vi "output.vi"() -> ()   [LabVIEW 2019]
uses:
  <vilib>/Rock Robotics/WPI/ThirdParty/Phoenix-LabVIEW/Motor Controller/Controls/CTRE_Phoenix_MotorControl_ControlMode.ctl
  <vilib>/Rock Robotics/WPI/Utilities/WPI_GetSetVariantRefNum.vi
  <vilib>/Rock Robotics/Network Tables/NT Write Boolean Array.vi
  <vilib>/Rock Robotics/Network Tables/NT Write Numeric Array.vi
panel:
  in  "Output 5":T1 items=["PercentOutput"=0, "Position"=1, "Velocity"=2, "Current"=3, "Follower"=5, "MotionProfile"=6, "MotionMagic"=7, "MotionProfileArc"=10, "Disabled"=15]
  in  "Intake 4":T1 items=["PercentOutput"=0, "Position"=1, "Velocity"=2, "Current"=3, "Follower"=5, "MotionProfile"=6, "MotionMagic"=7, "MotionProfileArc"=10, "Disabled"=15]
  in  "Intake 3":T1 items=["PercentOutput"=0, "Position"=1, "Velocity"=2, "Current"=3, "Follower"=5, "MotionProfile"=6, "MotionMagic"=7, "MotionProfileArc"=10, "Disabled"=15]
  in  "Output 4":T1 items=["PercentOutput"=0, "Position"=1, "Velocity"=2, "Current"=3, "Follower"=5, "MotionProfile"=6, "MotionMagic"=7, "MotionProfileArc"=10, "Disabled"=15]
  in  "Output 3":T1 items=["PercentOutput"=0, "Position"=1, "Velocity"=2, "Current"=3, "Follower"=5, "MotionProfile"=6, "MotionMagic"=7, "MotionProfileArc"=10, "Disabled"=15]
  in  "Intake 2":T1 items=["PercentOutput"=0, "Position"=1, "Velocity"=2, "Current"=3, "Follower"=5, "MotionProfile"=6, "MotionMagic"=7, "MotionProfileArc"=10, "Disabled"=15]
  in  "Intake":T1 items=["PercentOutput"=0, "Position"=1, "Velocity"=2, "Current"=3, "Follower"=5, "MotionProfile"=6, "MotionMagic"=7, "MotionProfileArc"=10, "Disabled"=15]
  in  "Output":T1 items=["PercentOutput"=0, "Position"=1, "Velocity"=2, "Current"=3, "Follower"=5, "MotionProfile"=6, "MotionMagic"=7, "MotionProfileArc"=10, "Disabled"=15]
  in  "Intake":T1 items=["PercentOutput"=0, "Position"=1, "Velocity"=2, "Current"=3, "Follower"=5, "MotionProfile"=6, "MotionMagic"=7, "MotionProfileArc"=10, "Disabled"=15]
  in  "Output":T1 items=["PercentOutput"=0, "Position"=1, "Velocity"=2, "Current"=3, "Follower"=5, "MotionProfile"=6, "MotionMagic"=7, "MotionProfileArc"=10, "Disabled"=15]
  in  "Intake":T1 items=["PercentOutput"=0, "Position"=1, "Velocity"=2, "Current"=3, "Follower"=5, "MotionProfile"=6, "MotionMagic"=7, "MotionProfileArc"=10, "Disabled"=15]
  in  "Output 2":T1 items=["PercentOutput"=0, "Position"=1, "Velocity"=2, "Current"=3, "Follower"=5, "MotionProfile"=6, "MotionMagic"=7, "MotionProfileArc"=10, "Disabled"=15]
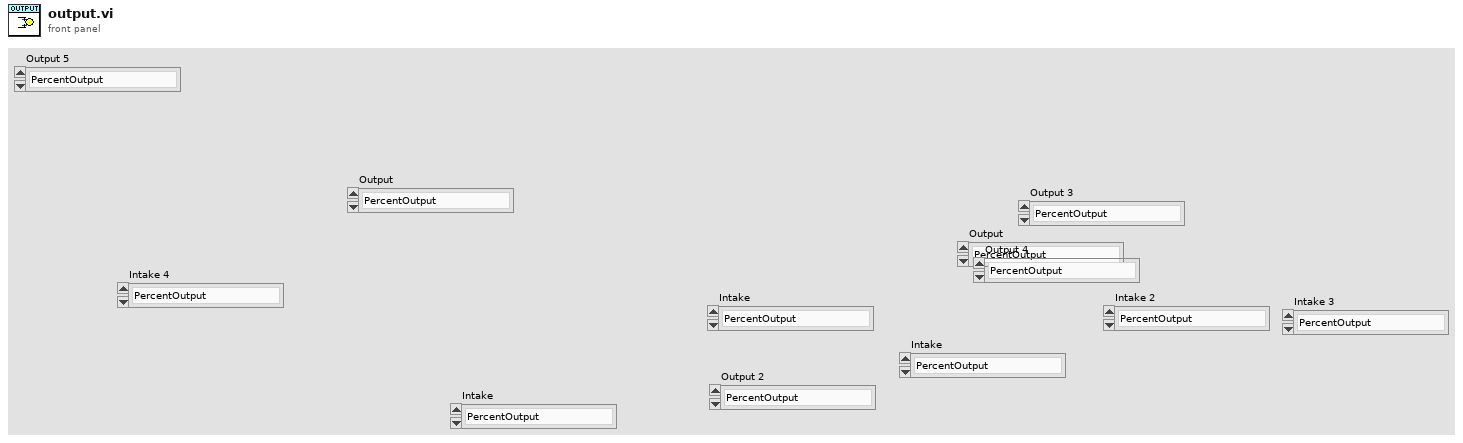
[diagram p1: front panel]
types:
  T1 = typedef "CTRE_Phoenix_MotorControl_ControlMode.ctl" = u16
  T2 = typedef "WPI_MotorControlDeviceRef.ctl" = cluster{"DeviceStatus":errorcluster, "Type":T3, "PWM":cluster{"PWM Channel":T4, "DeadBand":T5}, "CAN":cluster{"Device Number":u8, "SetOutput VI Ref":variant, "GetOutput VI Ref":variant, "Enable VI Ref":variant, "Disable VI Ref":variant, "Data":variant}, "Invert":bool, "DIO PWM":cluster{"PWM \"Enable\" Channel":T4, "DIOChannel":T6, "PWM Rate":dbl}}
  T3 = typedef "WPI_MotorControlType.ctl" = enum16{"PWM", "CAN", "DIO PWM"}
  T4 = typedef "FPGA_DIOPWMChannel.ctl" = enum8{"PWM 0", "PWM 1", "PWM 2", "PWM 3", "PWM 4", "PWM 5", "PWM 6", "PWM 7", "PWM 8", "PWM 9", "PWM MXP 0", "PWM MXP 1", "PWM MXP 2", "PWM MXP 3", "PWM MXP 4", "PWM MXP 5", "PWM MXP 6", "PWM MXP 7", "PWM MXP 8", "PWM MXP 9", "Invalid"}
  T5 = typedef "WPI_PWMDeadband.ctl" = cluster{"Name":string, "maxPositivePwm":i32, "minPositivePwm":i32, "centerPwm":i32, "maxNegativePwm":i32, "minNegativePwm":i32, "angularRange":u16}
  T6 = typedef "FPGA_DIOChannel.ctl" = enum8{"DIO 0", "DIO 1", "DIO 2", "DIO 3", "DIO 4", "DIO 5", "DIO 6", "DIO 7", "DIO 8", "DIO 9", "DIO MXP 0", "DIO MXP 1", "DIO MXP 2", "DIO MXP 3", "DIO MXP 4", "DIO MXP 5", "DIO MXP 6", "DIO MXP 7", "DIO MXP 8", "DIO MXP 9", "DIO MXP 10", "DIO MXP 11", "DIO MXP 12", "DIO MXP 13", "DIO MXP 14", "DIO MXP 15", "SPI Port CS1", "SPI Port CS2", "SPI Port CS3", "SPI Port MISO", "SPI Port MOSI", "Invalid"}
  T7 = typedef "WPI_JoystickDevRef.ctl" = cluster{"Device":T8}
  T8 = typedef "WPI_JoystickDeviceEnum.ctl" = enum16{"USB 0", "USB 1", "USB 2", "USB 3", "USB 4", "USB 5"}
  T9 = enum16{"Output Motor On", "Intake Motor On", "Complete"}
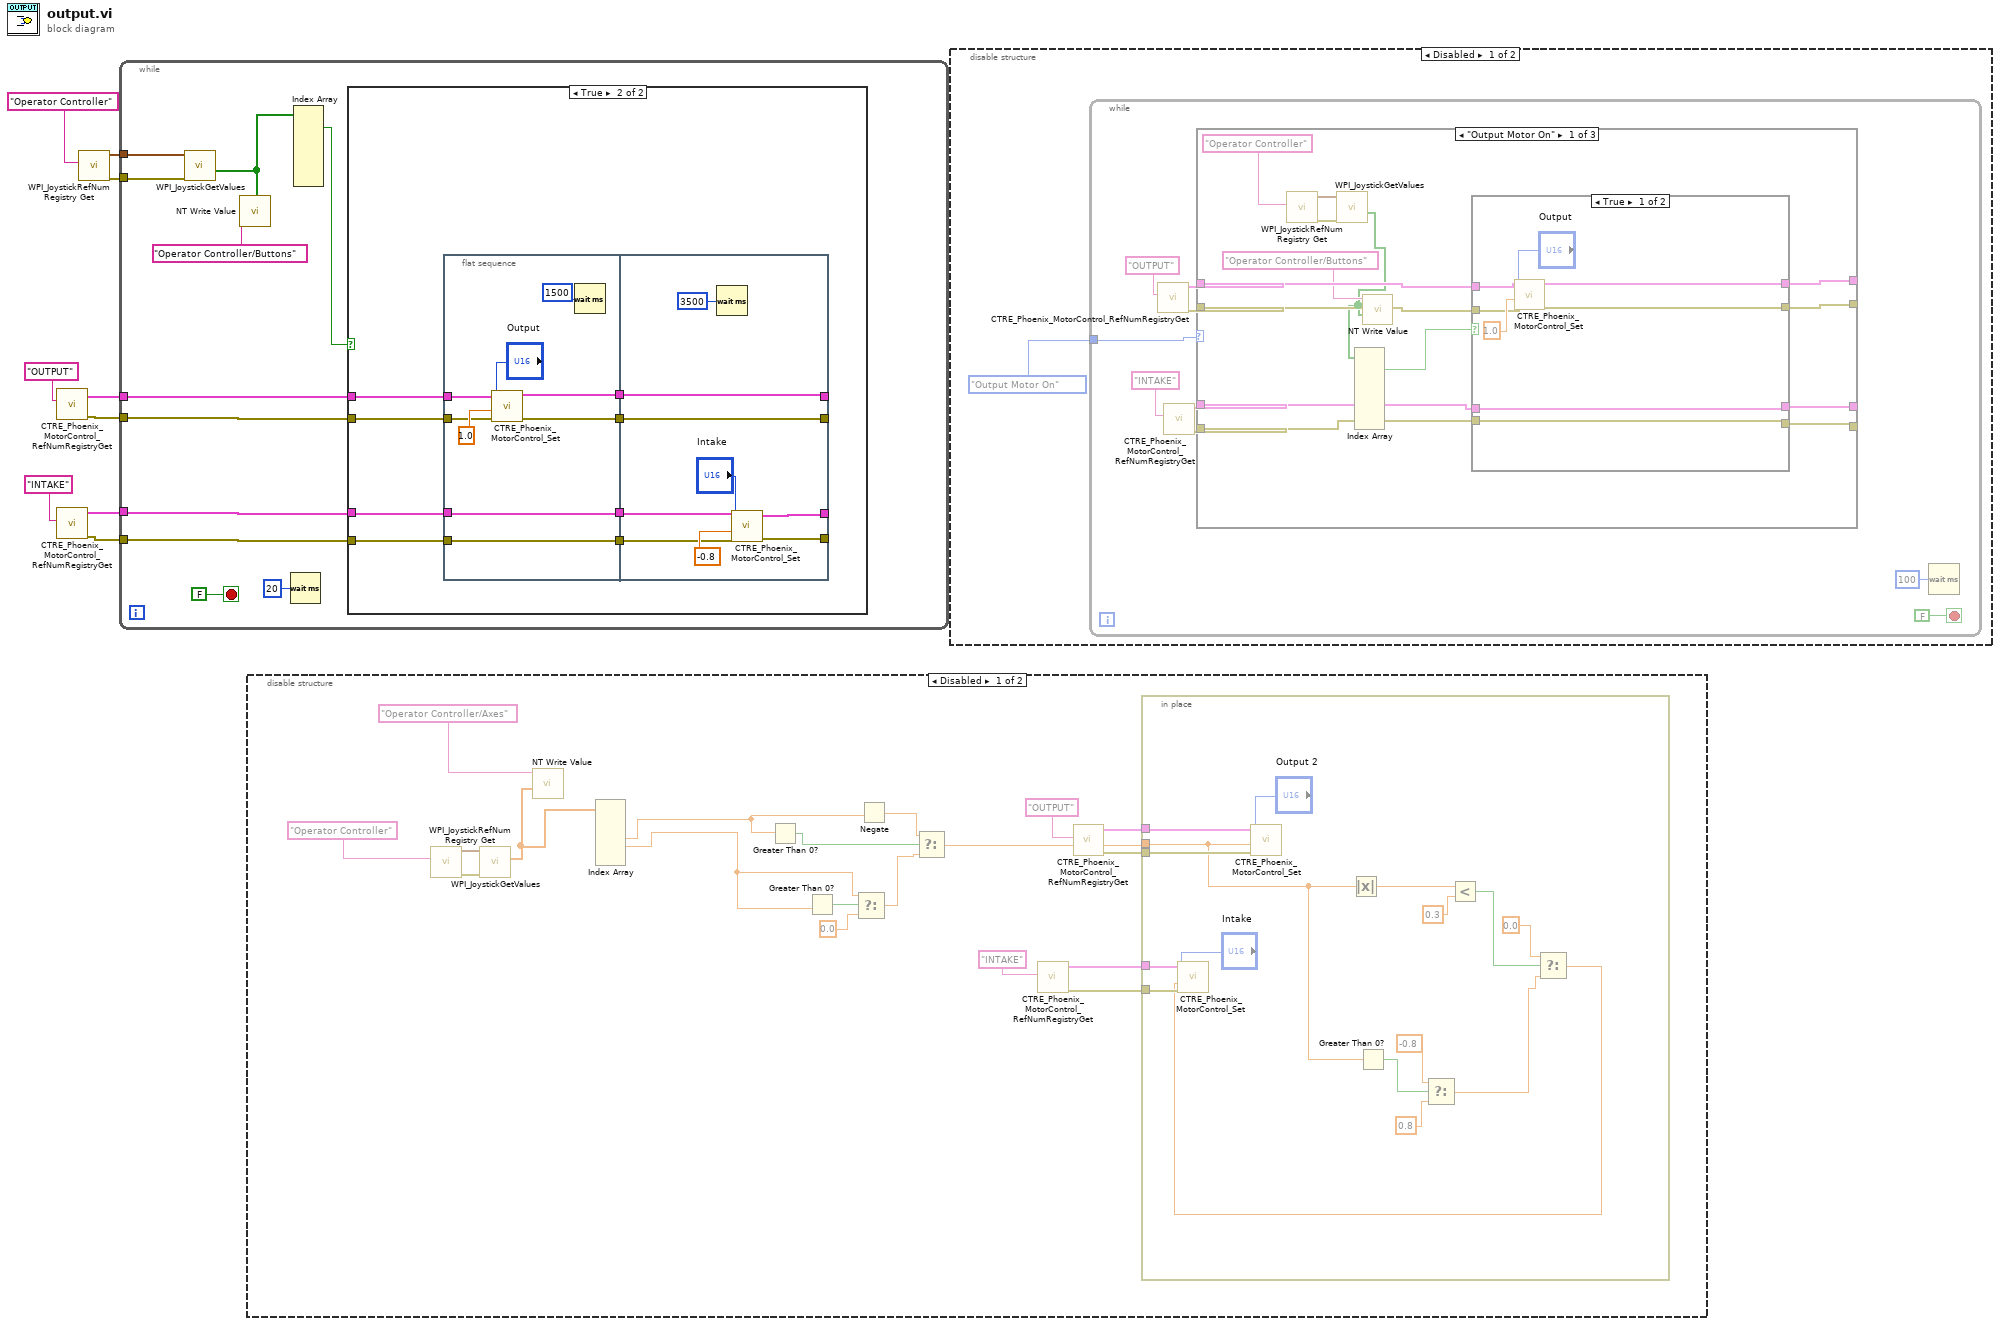
[diagram p0: block diagram]
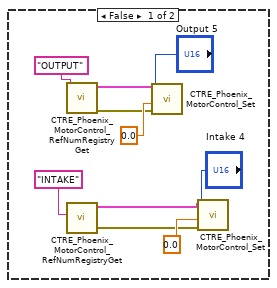
[diagram p2: hidden frame]
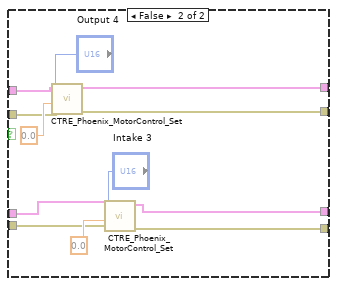
[diagram p3: hidden frame]
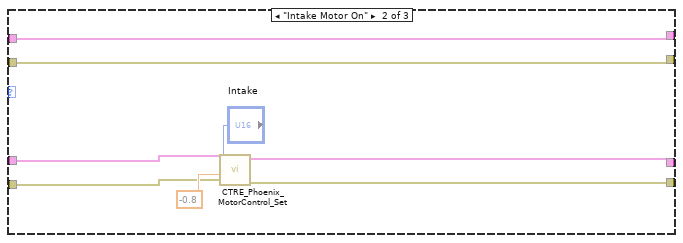
[diagram p4: hidden frame]
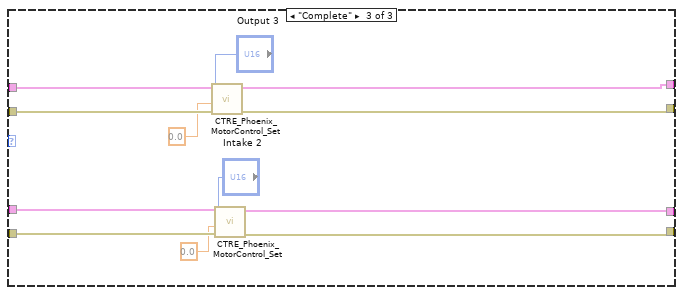
[diagram p5: hidden frame]
diagram:
  n1 = call <vilib>:"CTRE_Phoenix_MotorControl_RefNumRegistryGet.vi"("refnum name"="OUTPUT") -> ("error out"=w2:errorcluster, "PhoenixMotorControlDevRef"=w1:T2)  [unwired: 9 in]
  n2 = call <vilib>:"CTRE_Phoenix_MotorControl_RefNumRegistryGet.vi"("refnum name"="INTAKE") -> ("error out"=w4:errorcluster, "PhoenixMotorControlDevRef"=w3:T2)  [unwired: 9 in]
  n3 = call <vilib>:"WPI_JoystickRefNum Registry Get.vi"("refnum name"="Operator Controller") -> ("error out"=w7:errorcluster, "JoystickDevRef"=w8:T7)  [unwired: 1 in, 8 out]
  n4 = while {
    tunnel: w8 -> [w20]
    tunnel: w7 -> [w19]
    tunnel: w4 -> [w15]
    tunnel: w3 -> [w14]
    tunnel: w2 -> [w13]
    tunnel: w1 -> [w12]
    stop <- FALSE stop-if-true
    n5 = call <vilib>:"WPI_JoystickGetValues.vi"("error in (no error)"=w19, "JoystickDevRef"=w20) -> ("Buttons"=w17:bool[])  [unwired: 5 in, 4 out]
    n6 = call-poly <vilib>:"NT Write Value.vi"("Boolean Array"=w17, "Name"="Operator Controller/Buttons") -> ()  [unwired: 9 in, 1 out]
    n7 = Wait (ms)(milliseconds to wait=u32 20) -> ()  [unwired: 1 out]
    n8 = Index Array(array=w17) -> (element #1=w16:bool)  [unwired: 8 in, 7 out]
    n9 = case shown="True" w16 {
      tunnel: w15 -> [_ w34]
      tunnel: w14 -> [_ w33]
      tunnel: w13 -> [_ w32]
      tunnel: w12 -> [_ w31]
      frame False {
        n10 = call <vilib>:"CTRE_Phoenix_MotorControl_RefNumRegistryGet.vi"("refnum name"="OUTPUT") -> ("error out"=w23:errorcluster, "PhoenixMotorControlDevRef"=w24:T2)  [unwired: 9 in]
        n11 = call <vilib>:"CTRE_Phoenix_MotorControl_RefNumRegistryGet.vi"("refnum name"="INTAKE") -> ("error out"=w21:errorcluster, "PhoenixMotorControlDevRef"=w22:T2)  [unwired: 9 in]
        n12 = call <vilib>:"CTRE_Phoenix_MotorControl_Set.vi"("error in (no error)"=w23, "Output"=0.0, "Control Mode"="Output 5", "PhoenixMotorControlDevRef"=w24) -> ()  [unwired: 6 in, 2 out]
        n13 = call <vilib>:"CTRE_Phoenix_MotorControl_Set.vi"("error in (no error)"=w21, "Output"=0.0, "Control Mode"="Intake 4", "PhoenixMotorControlDevRef"=w22) -> ()  [unwired: 6 in, 2 out]
      }
      frame True {
        n14 = flat-sequence {
          tunnel: [w41] -> w38
          tunnel: [w42] -> w37
          tunnel: [w44] -> w36
          tunnel: [w43] -> w35
          tunnel: w34 -> [w42]
          tunnel: w33 -> [w41]
          tunnel: w32 -> [w40]
          tunnel: w31 -> [w39]
          tunnel: w38 -> [w53]
          tunnel: [w52] -> _
          tunnel: w37 -> [w51]
          tunnel: [w50] -> _
          tunnel: [w49] -> _
          tunnel: w36 -> [w49]
          tunnel: [w48] -> _
          tunnel: w35 -> [w48]
          frame #0 {
            n15 = call <vilib>:"CTRE_Phoenix_MotorControl_Set.vi"("error in (no error)"=w40, "Output"=1.0, "Control Mode"="Output", "PhoenixMotorControlDevRef"=w39) -> ("error out"=w44:errorcluster, "PhoenixMotorControlDevRef"=w43:T2)  [unwired: 6 in]
            n16 = Wait (ms)(milliseconds to wait=u32 1500) -> ()  [unwired: 1 out]
          }
          frame #1 {
            n17 = Wait (ms)(milliseconds to wait=u32 3500) -> ()  [unwired: 1 out]
            n18 = call <vilib>:"CTRE_Phoenix_MotorControl_Set.vi"("error in (no error)"=w51, "Output"=-0.8, "Control Mode"="Intake", "PhoenixMotorControlDevRef"=w53) -> ("error out"=w50:errorcluster, "PhoenixMotorControlDevRef"=w52:T2)  [unwired: 6 in]
          }
        }
      }
    }
  }
  n19 = disable-structure shown="Disabled" {
    frame Disabled {
      n20 = call <vilib>:"WPI_JoystickRefNum Registry Get.vi"("refnum name"="Operator Controller") -> ("error out"=w65:errorcluster, "JoystickDevRef"=w74:T7)  [unwired: 1 in, 8 out]
      n21 = call <vilib>:"WPI_JoystickGetValues.vi"("error in (no error)"=w65, "JoystickDevRef"=w74) -> ("Axes"=w66:dbl[])  [unwired: 5 in, 4 out]
      n22 = call-poly <vilib>:"NT Write Value.vi"("Numeric Array"=w66, "Name"="Operator Controller/Axes") -> ()  [unwired: 9 in, 1 out]
      n23 = Index Array(array=w66) -> (element #3=w64:dbl, element #4=w63:dbl)  [unwired: 6 in, 4 out]
      n24 = Greater Than 0?(x=w64) -> (x > 0?=w72:bool)
      n25 = Greater Than 0?(x=w63) -> (x > 0?=w70:bool)
      n26 = Select(t=w63, s=w70, f=0.0) -> (s? t:f=w68:dbl)
      n27 = Negate(x=w64) -> (-x=w71:dbl)
      n28 = Select(t=w71, s=w72, f=w68) -> (s? t:f=w60:dbl)
      n29 = call <vilib>:"CTRE_Phoenix_MotorControl_RefNumRegistryGet.vi"("refnum name"="INTAKE") -> ("error out"=w57:errorcluster, "PhoenixMotorControlDevRef"=w58:T2)  [unwired: 9 in]
      n30 = call <vilib>:"CTRE_Phoenix_MotorControl_RefNumRegistryGet.vi"("refnum name"="OUTPUT") -> ("error out"=w61:errorcluster, "PhoenixMotorControlDevRef"=w59:T2)  [unwired: 9 in]
      n31 = in-place {
        in-place-border: w61 -> [w90]
        in-place-border: w60 -> [w78]
        in-place-border: w59 -> [w89]
        in-place-border: w58 -> [w87]
        in-place-border: w57 -> [w86]
        n32 = call <vilib>:"CTRE_Phoenix_MotorControl_Set.vi"("error in (no error)"=w90, "Output"=w78, "Control Mode"="Output 2", "PhoenixMotorControlDevRef"=w89) -> ()  [unwired: 6 in, 2 out]
        n33 = Absolute Value(x=w78) -> (abs(x)=w82:dbl)
        n34 = Greater Than 0?(x=w78) -> (x > 0?=w85:bool)
        n35 = Select(t=-0.8, s=w85, f=0.8) -> (s? t:f=w77:dbl)
        n36 = Less?(x=w82, y=0.3) -> (x < y?=w80:bool)
        n37 = Select(t=0.0, s=w80, f=w77) -> (s? t:f=w76:dbl)
        n38 = call <vilib>:"CTRE_Phoenix_MotorControl_Set.vi"("error in (no error)"=w86, "Output"=w76, "Control Mode"="Intake", "PhoenixMotorControlDevRef"=w87) -> ()  [unwired: 6 in, 2 out]
      }
    }
    frame Enabled {
    }
  }
  n39 = disable-structure shown="Disabled" {
    frame Disabled {
      n40 = while {
        tunnel: T9."Output Motor On" -> [w93]
        stop <- FALSE stop-if-true
        n41 = call <vilib>:"CTRE_Phoenix_MotorControl_RefNumRegistryGet.vi"("refnum name"="OUTPUT") -> ("error out"=w98:errorcluster, "PhoenixMotorControlDevRef"=w99:T2)  [unwired: 9 in]
        n42 = call <vilib>:"CTRE_Phoenix_MotorControl_RefNumRegistryGet.vi"("refnum name"="INTAKE") -> ("error out"=w96:errorcluster, "PhoenixMotorControlDevRef"=w97:T2)  [unwired: 9 in]
        n43 = case shown="\"Output Motor On\"" w93 {
          tunnel: w99 -> [w115 w137 w148]
          tunnel: w98 -> [w114 w136 w147]
          tunnel: [w113 w137 w145] -> _
          tunnel: [w112 w136 w144] -> _
          tunnel: w97 -> [w109 w141 w152]
          tunnel: w96 -> [w108 w140 w154]
          tunnel: [w111 w139 w150] -> _
          tunnel: [w110 w138 w153] -> _
          frame "Output Motor On" {
            n44 = call <vilib>:"WPI_JoystickRefNum Registry Get.vi"("refnum name"="Operator Controller") -> ("error out"=w105:errorcluster, "JoystickDevRef"=w106:T7)  [unwired: 1 in, 8 out]
            n45 = call <vilib>:"WPI_JoystickGetValues.vi"("error in (no error)"=w105, "JoystickDevRef"=w106) -> ("Buttons"=w103:bool[])  [unwired: 5 in, 4 out]
            n46 = Index Array(array=w103) -> (element #1=w102:bool)  [unwired: 8 in, 7 out]
            n47 = call-poly <vilib>:"NT Write Value.vi"("Boolean Array"=w103, "Name"="Operator Controller/Buttons") -> ()  [unwired: 9 in, 1 out]
            n48 = case shown="True" w102 {
              tunnel: w115 -> [w121 w133]
              tunnel: w114 -> [w120 w132]
              tunnel: [w119 w131] -> w113
              tunnel: [w118 w130] -> w112
              tunnel: w109 -> [w117 w127]
              tunnel: w108 -> [w116 w126]
              tunnel: [w117 w125] -> w111
              tunnel: [w116 w124] -> w110
              frame True {
                n49 = call <vilib>:"CTRE_Phoenix_MotorControl_Set.vi"("error in (no error)"=w120, "Output"=1.0, "Control Mode"="Output", "PhoenixMotorControlDevRef"=w121) -> ("error out"=w118:errorcluster, "PhoenixMotorControlDevRef"=w119:T2)  [unwired: 6 in]
              }
              frame False {
                n50 = call <vilib>:"CTRE_Phoenix_MotorControl_Set.vi"("error in (no error)"=w132, "Output"=0.0, "Control Mode"="Output 4", "PhoenixMotorControlDevRef"=w133) -> ("error out"=w130:errorcluster, "PhoenixMotorControlDevRef"=w131:T2)  [unwired: 6 in]
                n51 = call <vilib>:"CTRE_Phoenix_MotorControl_Set.vi"("error in (no error)"=w126, "Output"=0.0, "Control Mode"="Intake 3", "PhoenixMotorControlDevRef"=w127) -> ("error out"=w124:errorcluster, "PhoenixMotorControlDevRef"=w125:T2)  [unwired: 6 in]
              }
            }
          }
          frame "Intake Motor On" {
            n52 = call <vilib>:"CTRE_Phoenix_MotorControl_Set.vi"("error in (no error)"=w140, "Output"=-0.8, "Control Mode"="Intake", "PhoenixMotorControlDevRef"=w141) -> ("error out"=w138:errorcluster, "PhoenixMotorControlDevRef"=w139:T2)  [unwired: 6 in]
          }
          frame "Complete" {
            n53 = call <vilib>:"CTRE_Phoenix_MotorControl_Set.vi"("error in (no error)"=w147, "Output"=0.0, "Control Mode"="Output 3", "PhoenixMotorControlDevRef"=w148) -> ("error out"=w144:errorcluster, "PhoenixMotorControlDevRef"=w145:T2)  [unwired: 6 in]
            n54 = call <vilib>:"CTRE_Phoenix_MotorControl_Set.vi"("error in (no error)"=w154, "Output"=0.0, "Control Mode"="Intake 2", "PhoenixMotorControlDevRef"=w152) -> ("error out"=w153:errorcluster, "PhoenixMotorControlDevRef"=w150:T2)  [unwired: 6 in]
          }
        }
        n55 = Wait (ms)(milliseconds to wait=u32 100) -> ()  [unwired: 1 out]
      }
    }
    frame Enabled {
    }
  }
